vi "sv_Fractional-octave Analysis with IC (linear mode).vi"(0 "scaled signal [EU]":dbl[](array[numeric]) format="%.2f", 1 "linear averaging mode":T1(ring), 2 "filter bank parameters":T2 {"standard filter bandwidth" format="%.2f"; "special filter bandwidth" format="%.2f"; "lowpass filter coefficients"."Forward Coefficients" format="%.2f"; "lowpass filter coefficients"."Reverse Coefficients" format="%.2f"; "standard filter coefficients"."Forward Coefficients" format="%.2f"; "standard filter coefficients"."Reverse Coefficients" format="%.2f"; "special filter coefficients"."Forward Coefficients" format="%.2f"; "special filter coefficients"."Reverse Coefficients" format="%.2f"}, 3 "internal filter state IN":T3 {"linear averaging"."size" format="%.2f"; "linear averaging"."squared sum" format="%.2f"; "exponential averaging"."peak detector" format="%.2f"; "exponential averaging"."exponential averaging" format="%.2f"; "result" format="%.2f"; "lowpass filter" format="%.2f"; "octave filter"."Octave filter" format="%.2f"}, 4 "reset averaging (F)":bool, 5 "filter init/cont (init:F)":bool) -> (6 "linear avg band power [EU^2 rms]":dbl[](array[numeric]) format="%.2f", 7 "settled?":bool, 8 "internal filter state OUT":T3 {"linear averaging"."size" format="%.2f"; "linear averaging"."squared sum" format="%.2f"; "exponential averaging"."peak detector" format="%.2f"; "exponential averaging"."exponential averaging" format="%.2f"; "result" format="%.2f"; "lowpass filter" format="%.2f"; "octave filter"."Octave filter" format="%.2f"})   [LabVIEW 2017, in "SoundVib_Octave.lvlib"]
doc: "Performs a linear average fractional-octave analysis on the input signal. This VI requires the filter bank parameters and initialize filter state information the Design Octave Filter Set VI generates.\nThis VI returns the linear average power in each fractional-octave band.\nThe internal filter state IN and internal filter state OUT keep track of the internal state of the filter to ensure continuous operation of the filter. To achieve this continuous operation, you must call this VI the first time with filter init/cont set to FALSE. Call it all subsequent times with filter init/cont set to TRUE. Wire the internal filter state OUT of this call to the internal filter state IN for the next call to this VI."
uses:
  <vilib>/addons/Sound and Vibration/svt_Octave/SoundVib_Octave.lvlib
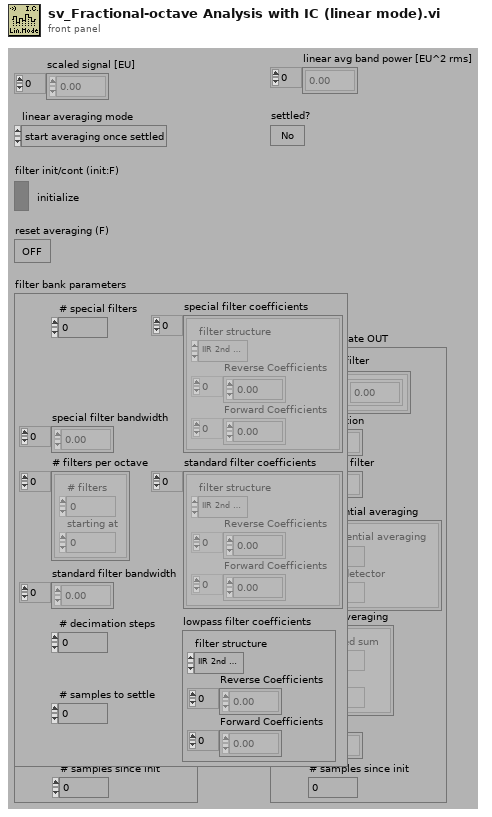
[diagram p1: front panel]
types:
  T1 = enum16{"start averaging once settled", "continuous averaging", "single averaging"}
  T2 = cluster{"# special filters":i32, "special filter coefficients":cluster{"filter structure":enum32{"IIR 2nd Order", "IIR 4th Order"}, "Reverse Coefficients":dbl[], "Forward Coefficients":dbl[]}[], "# filters per octave":cluster{"# filters":i32, "starting at":i32}[], "standard filter coefficients":cluster{"filter structure":enum32{"IIR 2nd Order", "IIR 4th Order"}, "Reverse Coefficients":dbl[], "Forward Coefficients":dbl[]}[], "# decimation steps":i32, "lowpass filter coefficients":cluster{"filter structure":enum32{"IIR 2nd Order", "IIR 4th Order"}, "Reverse Coefficients":dbl[], "Forward Coefficients":dbl[]}, "# samples to settle":u64, "special filter bandwidth":dbl[], "standard filter bandwidth":dbl[]}
  T3 = cluster{"octave filter":cluster{"Octave filter":dbl[]}[], "decimation":i32[], "lowpass filter":dbl[][], "exponential averaging":cluster{"exponential averaging":dbl, "peak detector":dbl}[], "linear averaging":cluster{"squared sum":dbl, "size":dbl}[], "result":dbl[], "# samples since init":u64}
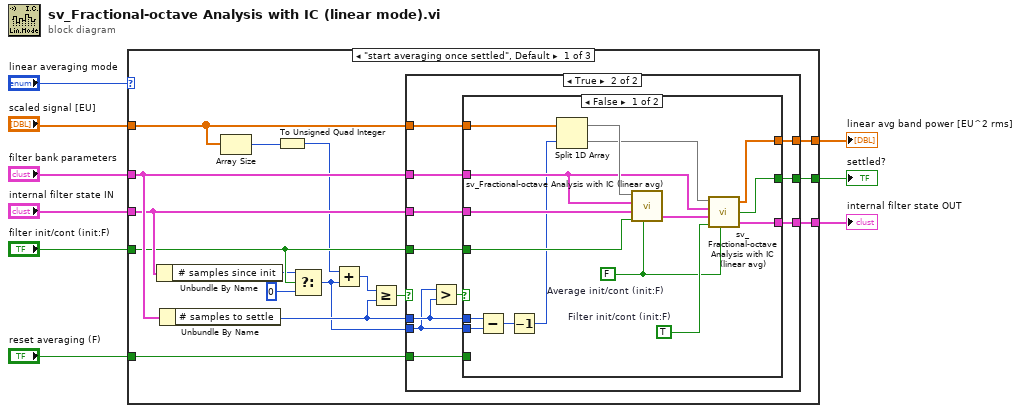
[diagram p0: block diagram]
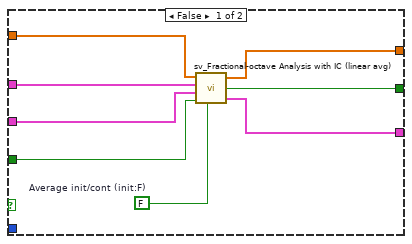
[diagram p2: hidden frame]
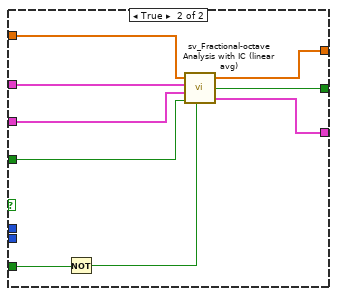
[diagram p3: hidden frame]
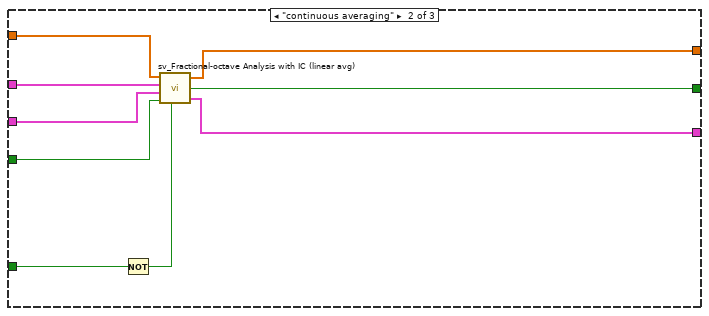
[diagram p4: hidden frame]
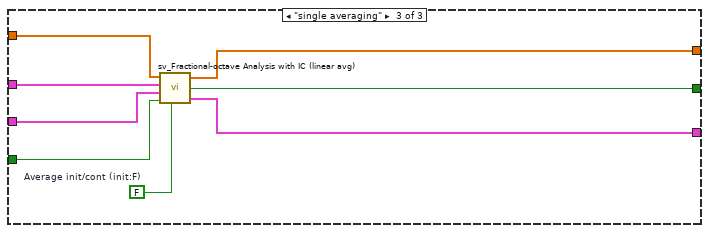
[diagram p5: hidden frame]
diagram:
  n1 = case shown="\"start averaging once settled\", Default" "linear averaging mode" {
    tunnel: "scaled signal [EU]" -> [w19 w78 w86]
    tunnel: "filter bank parameters" -> [w25 w77 w85]
    tunnel: "internal filter state IN" -> [w24 w76 w84]
    tunnel: "filter init/cont (init:F)" -> [w21 w75 w83]
    tunnel: [w14 w74 w81] -> w4
    tunnel: [w13 w73 w80] -> w3
    tunnel: [w12 w72 w79] -> w2
    tunnel: "reset averaging (F)" -> [w11 w71 _]
    frame "start averaging once settled", Default {
      n2 = Unbundle By Name(w24) -> ("# samples since init"=w20:u64)
      n3 = Unbundle By Name(w25) -> ("# samples to settle"=w23:u64)
      n4 = Array Size(array=w19) -> (size(s)=w17:i32)
      n5 = To Unsigned Quad Integer(1:w17) -> (0:w10:u64)
      n6 = Select(t=w20, s=w21, f=u64 0) -> (s? t:f=w15:u64)
      n7 = Add(x=w10, y=w15) -> (x+y=w16:u64)
      n8 = Greater Or Equal?(x=w16, y=w23) -> (x >= y?=w22:bool)
      n9 = case shown="True" w22 {
        tunnel: w25 -> [w33 w44]
        tunnel: w19 -> [w32 w41]
        tunnel: w24 -> [w30 w43]
        tunnel: w21 -> [w29 w42]
        tunnel: w23 -> [_ w39]
        tunnel: w15 -> [_ w38]
        tunnel: [w28 w37] -> w14
        tunnel: [w27 w36] -> w13
        tunnel: [w26 w35] -> w12
        tunnel: w11 -> [_ w34]
        frame False {
          w31 = FALSE  # Average init/cont (init:F)
          n10 = call <vilib>:"sv_Fractional-octave Analysis with IC (linear avg).vi"("scaled signal [EU]"=w32, "filter bank parameters"=w33, "internal filter state IN"=w30, "average init/cont (cont:T)"=w31, "filter init/cont (init:F)"=w29) -> ("linear avg band power [EU^2 rms]"=w28:dbl[], "settled?"=w27:bool, "internal filter state OUT"=w26:T3)  [unwired: 1 in]
        }
        frame True {
          n11 = Greater?(x=w38, y=w39) -> (0:w40:bool)
          n12 = case shown="False" w40 {
            tunnel: w44 -> [w50 w69]
            tunnel: w43 -> [w55 w68]
            tunnel: w42 -> [w54 w67]
            tunnel: w41 -> [w60 w66]
            tunnel: w39 -> [w59 _]
            tunnel: w38 -> [w58 _]
            tunnel: [w48 w65] -> w37
            tunnel: [w47 w64] -> w36
            tunnel: [w46 w63] -> w35
            tunnel: w34 -> [_ w62]
            frame False {
              w53 = TRUE  # Filter init/cont (init:F)
              w49 = FALSE  # Average init/cont (init:F)
              n13 = Subtract(x=w59, y=w58) -> (x-y=w57:u64)
              n14 = Decrement(x=w57) -> (x-1=w45:u64)
              n15 = Split 1D Array(array=w60, index=w45) -> (first subarray=w56:dbl[], second subarray=w52:dbl[])
              n16 = call <vilib>:"sv_Fractional-octave Analysis with IC (linear avg).vi"("scaled signal [EU]"=w56, "filter bank parameters"=w50, "internal filter state IN"=w55, "average init/cont (cont:T)"=w49, "filter init/cont (init:F)"=w54) -> ("internal filter state OUT"=w51:T3)  [unwired: 1 in, 2 out]
              n17 = call <vilib>:"sv_Fractional-octave Analysis with IC (linear avg).vi"("scaled signal [EU]"=w52, "filter bank parameters"=w50, "internal filter state IN"=w51, "average init/cont (cont:T)"=w49, "filter init/cont (init:F)"=w53) -> ("linear avg band power [EU^2 rms]"=w48:dbl[], "settled?"=w47:bool, "internal filter state OUT"=w46:T3)  [unwired: 1 in]
            }
            frame True {
              n18 = Not(x=w62) -> (.not. x?=w61:bool)
              n19 = call <vilib>:"sv_Fractional-octave Analysis with IC (linear avg).vi"("scaled signal [EU]"=w66, "filter bank parameters"=w69, "internal filter state IN"=w68, "average init/cont (cont:T)"=w61, "filter init/cont (init:F)"=w67) -> ("linear avg band power [EU^2 rms]"=w65:dbl[], "settled?"=w64:bool, "internal filter state OUT"=w63:T3)  [unwired: 1 in]
            }
          }
        }
      }
    }
    frame "continuous averaging" {
      n20 = Not(x=w71) -> (.not. x?=w70:bool)
      n21 = call <vilib>:"sv_Fractional-octave Analysis with IC (linear avg).vi"("scaled signal [EU]"=w78, "filter bank parameters"=w77, "internal filter state IN"=w76, "average init/cont (cont:T)"=w70, "filter init/cont (init:F)"=w75) -> ("linear avg band power [EU^2 rms]"=w74:dbl[], "settled?"=w73:bool, "internal filter state OUT"=w72:T3)  [unwired: 1 in]
    }
    frame "single averaging" {
      w82 = FALSE  # Average init/cont (init:F)
      n22 = call <vilib>:"sv_Fractional-octave Analysis with IC (linear avg).vi"("scaled signal [EU]"=w86, "filter bank parameters"=w85, "internal filter state IN"=w84, "average init/cont (cont:T)"=w82, "filter init/cont (init:F)"=w83) -> ("linear avg band power [EU^2 rms]"=w81:dbl[], "settled?"=w80:bool, "internal filter state OUT"=w79:T3)  [unwired: 1 in]
    }
  }
  "linear avg band power [EU^2 rms]" <- w4
  "internal filter state OUT" <- w2
  "settled?" <- w3
